vi "object_tracking_subVI_2.vi"(0 "ROI Descriptor (Image Mask 1)":T2={"Global Rectangle"=[272, 198, 466, 320], "Contours"=[{"ID"=enum."External", "Type"=3, "Coordinates"=[272, 198, 466, 320]}]} {"Contours"."Type" items=["No Selection", "Point", "Line", "Rectangle", "Oval", "Polygon", "Freehand Region", "Annulus", "Unused2", "Unused3", "Broken Line", "Freehand Line", "Rotated Rectangle"]}, 1 "Image":T1, 7 "error in":errorcluster) -> (20 "Objects (pixel) (Object Tracking 1)":T3(array[cluster]), 21 "Image Out":T1(plugin-control), 27 "error out":errorcluster)   [LabVIEW 2024]
doc: "Este subVI realiza el procesado de las imágenes capturadas en tiempo real. Contiene el proceso de adquisición, image mask, color plane extraction, gray morphological y object tracking.\n\nAutores:\nIvan Nieto Guerrero, David Alejandro Zarazúa Martínez\n\n06/Mar/2025"
uses:
  <vilib>/vision/Image Controls.llb/IMAQ Image.ctl
  <vilib>/vision/Tracking.llb/IMAQ Object Tracking SessionType.ctl
  <vilib>/vision/Vision Assistant Utils.llb/IVA Object Tracking - Init Function.ctl
  <vilib>/vision/NI_Vision_Development_Module.lvlib
panel:
  in  "error in (no error)":errorcluster
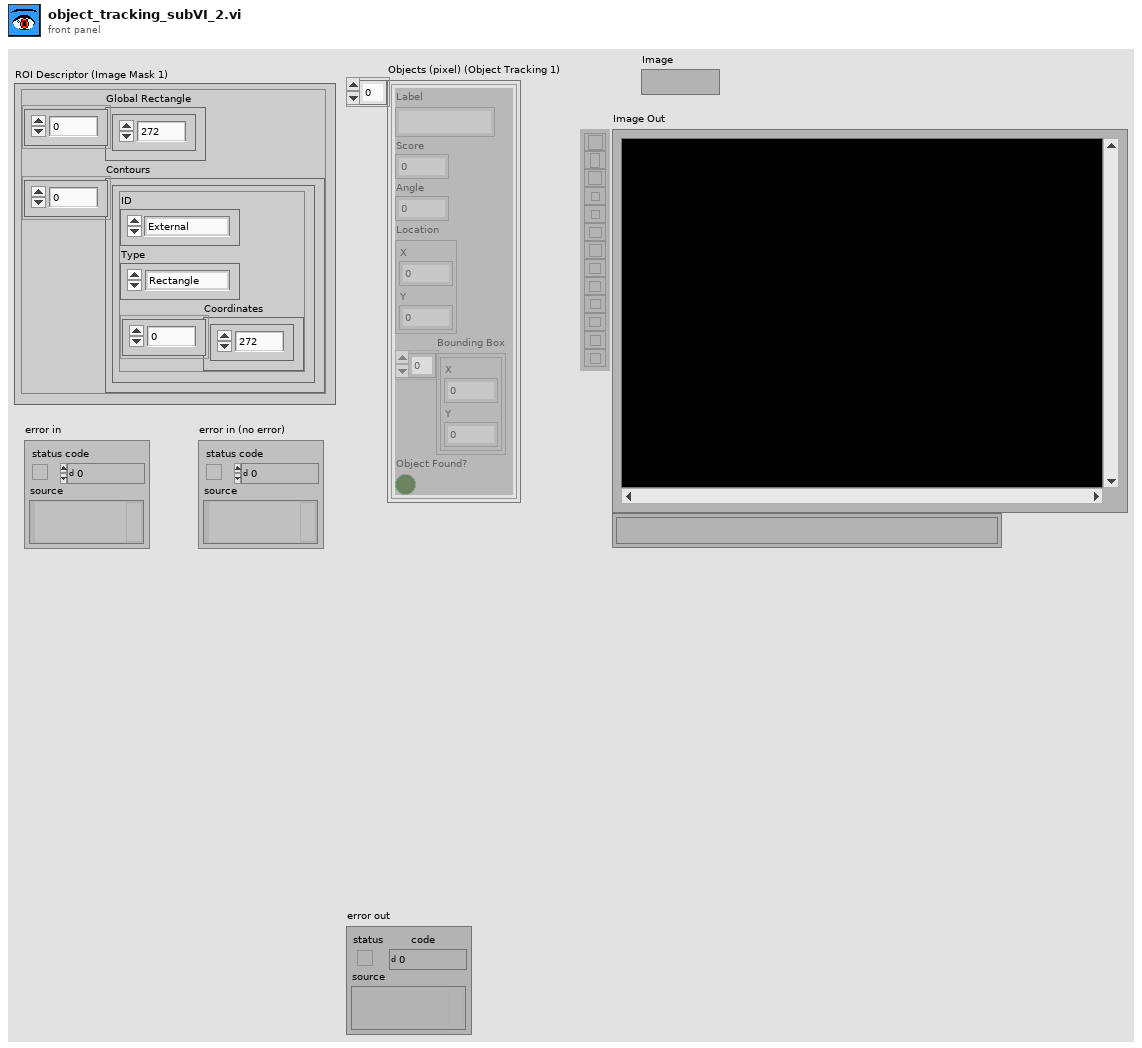
[diagram p1: front panel]
types:
  T1 = typedef "IMAQ Image.ctl" = refnum<image>
  T2 = cluster{"Global Rectangle":i32[], "Contours":cluster{"ID":enum32{"External", "Internal"}, "Type":u32, "Coordinates":i32[]}[]}
  T3 = cluster{"Label":string, "Score":i32, "Angle":dbl, "Location":cluster{"X":dbl, "Y":dbl}, "Bounding Box":cluster{"X":dbl, "Y":dbl}[], "Object Found?":bool}[]
  T4 = cluster{"Number of Histogram Bins":i32, "Blending Parameter (%)":dbl, "Max Scale Change (%)":dbl, "Max Rotation Change":dbl, "Max Shape Change (%)":dbl, "Maximum Iterations":i32}
  T5 = typedef "IVA Object Tracking - Init Function.ctl" = enum16{"Init", "Get", "Set"}
  T6 = cluster{"Initial Position":cluster{"Source":enum16{"Constant", "Measure"}, "Point ID":cluster{"GUID":string, "Index":i32}, "Point":cluster{"x":sgl, "y":sgl}}, "Initial Angle":cluster{"Source":enum16{"Constant", "Measure"}, "Measure ID":cluster{"GUID":string, "Index":i32}, "Value":dbl}}[]
  T7 = typedef "IMAQ Object Tracking SessionType.ctl" = i32
  T8 = enum32{"AutoM", "Close", "Dilate", "Erode", "Gradient", "Gradient in", "Gradient out", "HitMiss", "Open", "PClose", "POpen", "Thick", "Thin"}
  T9 = typedef "Image Type" = u32
  T10 = cluster{"Number of Histogram Bins":i32, "Blending Parameter (%)":dbl, "Maximum Iterations":i32}
  T11 = typedef "IMAQ Object Tracking Session.ctl" = refnum<k20>
  T12 = cluster{"Source":enum16{"Constant", "Measure"}, "Point ID":cluster{"GUID":string, "Index":i32}, "Point":cluster{"x":sgl, "y":sgl}}
  T13 = cluster{"Source":enum16{"Constant", "Measure"}, "Measure ID":cluster{"GUID":string, "Index":i32}, "Value":dbl}
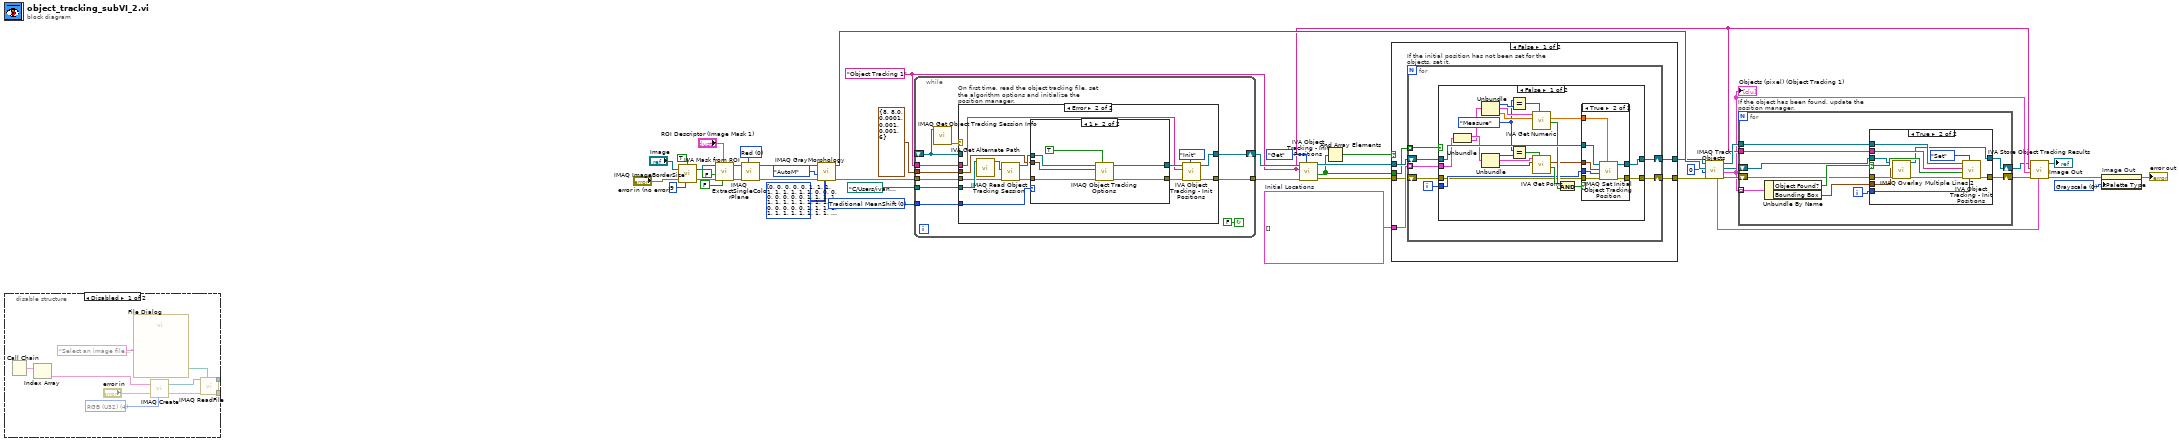
[diagram p0: block diagram]
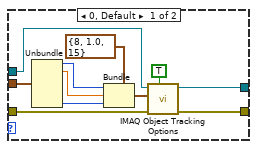
[diagram p8: hidden frame]
diagram:
  w4 = u32 0 items=["Grayscale", "Binary", "Gradient", "Rainbow", "Temperature", "User Defined", "Binary 16 Bit", "Gradient 16 Bit", "Rainbow 16 Bit", "Temperature 16 Bit", "User Defined 16 Bit"] ("Palette Type")
  w12 = "Object Tracking 1" ("Step Name")
  w26 = T6 []  # Initial Locations
  w28 = T7 0 items=["Traditional MeanShift", "Shape Adapted MeanShift"] ("Algorithm")
  w36 = 0 items=["Red", "Green", "Blue", "Hue", "Saturation", "Luminance", "Value", "Intensity"] ("Color Plane")
  n1 = disable-structure shown="Disabled" {
    disable-tunnel: [w54 _] -> _
    disable-tunnel: [w45 _] -> _
    frame Disabled {
      w46 = T9 4 items=["Grayscale (U8)", "Grayscale (I16)", "Grayscale (SGL)", "Complex (CSG)", "RGB (U32)", "HSL (U32)", "RGB (U64)", "Grayscale (U16)"] ("Image Type")
      n2 = Call Chain() -> (call chain=w50:string[])
      n3 = Index Array(array=w50) -> (element=w49:string)  [unwired: 1 in]
      n4 = call "File Dialog"("prompt"="Select an image file...") -> ("selected path"=w47:path)  [unwired: 6 in, 8 out]
      n5 = call "IMAQ Create"("Image Name"=w49, "Image Type"=w46, "error in (no error)"="error in") -> ("New Image"=w53:T1, "error out"=w52:errorcluster)  [unwired: 1 in, 1 out]
      n6 = call "IMAQ ReadFile"("File Path"=w47, "error in (no error)"=w52, "Image"=w53) -> ("error out"=w54:errorcluster, "Image Out"=w45:T1)  [unwired: 2 in, 5 out]
    }
    frame Enabled {
    }
  }
  n7 = call "IMAQ ImageBorderSize"("Get/Set Status? (Set)"=TRUE, "Image"="Image", "Image border size in"=9 ("Border Size"), "error in (no error)"="error in (no error)") -> ("Image Out"=w39:T1, "error out"=w44:errorcluster)  [unwired: 1 out]
  n8 = call <vilib>:"IVA Mask from ROI.vi"("Shrink"=FALSE, "ROI Descriptor"="ROI Descriptor (Image Mask 1)", "error in (no error)"=w44, "Out / In"=FALSE, "Image Src"=w39) -> ("error out"=w37:errorcluster, "Image Out"=w35:T1)  [unwired: 5 out]
  n9 = call "IMAQ ExtractSingleColorPlane"("Color Plane"=w36, "error in (no error)"=w37, "Image Src"=w35) -> ("error out"=w34:errorcluster, "Image Dst Out"=w31:T1)  [unwired: 1 in, 6 out]
  n10 = call "IMAQ GrayMorphology"("Structuring Element"=i32[][] [[0, 0, 0, 0, 0, 1, 1, 1, 1, 1, 1, 1, 1, 1, 0, 0, 0, 0, 0], [0, 0, 0, 1, 1, 1, 1, 1, 1, 1, 1, 1, 1, 1, 1, 1, 0, 0, 0], [0, 0, 1, 1, 1, 1, 1, 1, 1, 1, 1, 1, 1, 1, 1, 1, 1, 0, 0], [0, 1, 1, 1, 1, 1, 1, 1, 1, 1, 1, 1, 1, 1, 1, 1, 1, 1, 0], [0, 1, 1, 1, 1, 1, 1, 1, 1, 1, 1, 1, 1, 1, 1, 1, 1, 1, 0], [1, 1, 1, 1, 1, 1, 1, 1, 1, 1, 1, 1, 1, 1, 1, 1, 1, 1, 1], [1, 1, 1, 1, 1, 1, 1, 1, 1, 1, 1, 1, 1, 1, 1, 1, 1, 1, 1], [1, 1, 1, 1, 1, 1, 1, 1, 1, 1, 1, 1, 1, 1, 1, 1, 1, 1, 1], [1, 1, 1, 1, 1, 1, 1, 1, 1, 1, 1, 1, 1, 1, 1, 1, 1, 1, 1], [1, 1, 1, 1, 1, 1, 1, 1, 1, 1, 1, 1, 1, 1, 1, 1, 1, 1, 1], [1, 1, 1, 1, 1, 1, 1, 1, 1, 1, 1, 1, 1, 1, 1, 1, 1, 1, 1], [1, 1, 1, 1, 1, 1, 1, 1, 1, 1, 1, 1, 1, 1, 1, 1, 1, 1, 1], [1, 1, 1, 1, 1, 1, 1, 1, 1, 1, 1, 1, 1, 1, 1, 1, 1, 1, 1], [1, 1, 1, 1, 1, 1, 1, 1, 1, 1, 1, 1, 1, 1, 1, 1, 1, 1, 1], [0, 1, 1, 1, 1, 1, 1, 1, 1, 1, 1, 1, 1, 1, 1, 1, 1, 1, 0], [0, 1, 1, 1, 1, 1, 1, 1, 1, 1, 1, 1, 1, 1, 1, 1, 1, 1, 0], [0, 0, 1, 1, 1, 1, 1, 1, 1, 1, 1, 1, 1, 1, 1, 1, 1, 0, 0], [0, 0, 0, 1, 1, 1, 1, 1, 1, 1, 1, 1, 1, 1, 1, 1, 0, 0, 0], [0, 0, 0, 0, 0, 1, 1, 1, 1, 1, 1, 1, 1, 1, 0, 0, 0, 0, 0]], "error in (no error)"=w34, "Operation"=T8."AutoM", "Image Src"=w31) -> ("error out"=w30:errorcluster, "Image Dst Out"=w29:T1)  [unwired: 3 in, 3 out]
  n11 = while {
    shift-right: [w64] -> w24
    shift-left: _ -> [w55]
    tunnel: path "C:/Users/ivanu/OneDrive/Escritorio/Universidad/Semestre 8/Instrumentacion/Proyecto Final_Eye_detection/pupila_1.nitf.png" ("Tracking Session File Path") -> [w62]
    tunnel: w30 -> [w61]
    tunnel: w28 -> [w60]
    tunnel: [w59] -> w21
    tunnel: T4 {"Number of Histogram Bins"=8, "Blending Parameter (%)"=8.0, "Max Scale Change (%)"=0.0001, "Max Rotation Change"=0.001, "Max Shape Change (%)"=0.001, "Maximum Iterations"=6} ("Options") -> [w58]
    tunnel: w12 -> [w57]
    stop <- FALSE continue-if-true
    n12 = call "IMAQ Get Object Tracking Session Info"("Object Tracking Session In"=w55) -> ("error out"=w56:errorcluster)  [unwired: 1 in, 9 out]
    n13 = case "On first time, read the object tracking file, set the algorithm options and initialize the position manager." shown="Error" w56 {
      tunnel: [w66 w71] -> w64
      tunnel: w55 -> [w66 _]
      tunnel: w62 -> [_ w79]
      tunnel: w61 -> [w65 w77]
      tunnel: w60 -> [_ w76]
      tunnel: [w65 w70] -> w59
      tunnel: w58 -> [_ w73]
      tunnel: w57 -> [_ w67]
      frame No Error {
      }
      frame Error {
        n14 = call <vilib>:"IVA Get Alternate Path.vi"("Path In"=w79) -> ("Path Out"=w78:path)  [unwired: 10 out]
        n15 = call "IMAQ Read Object Tracking Session"("error in (no error)"=w77, "Object Tracking Session File Path"=w78) -> ("error out"=w74:errorcluster, "Object Tracking Session Out"=w75:T11)  [unwired: 1 in, 7 out]
        n16 = case shown="1" w76 {
          tunnel: w75 -> [w90 w96]
          tunnel: [w89 w95] -> w72
          tunnel: w74 -> [w88 w94]
          tunnel: [w87 w93] -> w69
          tunnel: w73 -> [w86 w92]
          frame 0, Default {
            n17 = Unbundle(w86) -> ("Number of Histogram Bins"=w85:i32, "Blending Parameter (%)"=w84:dbl, "Maximum Iterations"=w80:i32)  [unwired: 3 out]
            n18 = Bundle(cluster=T10 {"Number of Histogram Bins"=8, "Blending Parameter (%)"=1.0, "Maximum Iterations"=15} ("Mean Shift Options in"), "Number of Histogram Bins"=w85, "Blending Parameter (%)"=w84, "Maximum Iterations"=w80) -> (w83:T10)
            n19 = call-poly "IMAQ Object Tracking Options"("Get/Set (Get)"=TRUE, "error in (no error)"=w88, "Mean Shift Options in"=w83, "Object Tracking Session In"=w90) -> ("error out"=w87:errorcluster, "Object Tracking Session Out"=w89:T11)  [unwired: 1 in, 5 out]
          }
          frame 1 {
            n20 = call-poly "IMAQ Object Tracking Options"("Get/Set (Get)"=TRUE, "error in (no error)"=w94, "Shape Adapted Options in"=w92, "Object Tracking Session In"=w96) -> ("error out"=w93:errorcluster, "Object Tracking Session Out"=w95:T11)  [unwired: 2 in, 4 out]
          }
        }
        n21 = call <vilib>:"IVA Object Tracking - Init Positions.vi"("Function"=IVA_Object_Tracking_-_Init_Function."Init", "error in (no error)"=w69, "Process ID"=w67, "Object Tracking Session In"=w72) -> ("error out"=w70:errorcluster, "Object Tracking Session dup"=w71:T11)  [unwired: 2 in, 4 out]
      }
    }
  }
  n22 = call <vilib>:"IVA Object Tracking - Init Positions.vi"("Function"=IVA_Object_Tracking_-_Init_Function."Get", "error in (no error)"=w21, "Process ID"=w12, "Object Tracking Session In"=w24) -> ("error out"=w20:errorcluster, "Init Values Out"=w18:bool[], "Object Tracking Session dup"=w23:T11)  [unwired: 2 in, 3 out]
  n23 = And Array Elements(Boolean array=w18) -> (logical AND=w19:bool)
  n24 = case shown="False" w19 {
    tunnel: w26 -> [w102 _]
    tunnel: [w101 w144] -> w25
    tunnel: w23 -> [w100 w144]
    tunnel: w20 -> [w99 w143]
    tunnel: w18 -> [w98 _]
    tunnel: [w97 w143] -> w17
    frame False {
      n25 = for "If the initial position has not been set for the objects, set it." {
        tunnel: w102 -> [w108] mode=indexing
        shift-right: [w106] -> w101
        shift-left: w100 -> [w109]
        shift-right: [w103] -> w97
        shift-left: w99 -> [w105]
        tunnel: w98 -> [w104] mode=indexing
        i -> [w107]
        n26 = case shown="False" w104 {
          tunnel: w109 -> [w131 w142]
          tunnel: w108 -> [w130 _]
          tunnel: w107 -> [w114 _]
          tunnel: [w112 w142] -> w106
          tunnel: w105 -> [w111 w141]
          tunnel: [w110 w141] -> w103
          frame False {
            w120 = enum16{"Constant", "Measure"}."Measure" ("Source")
            n27 = Unbundle(w130) -> ("Initial Position"=w129:T12, "Initial Angle"=w128:T13)
            n28 = Unbundle(w128) -> ("Source"=w121:enum16{"Constant", "Measure"}, "Measure ID"=w125:cluster{"GUID":string, "Index":i32}, "Value"=w124:dbl)
            n29 = Unbundle(w129) -> ("Source"=w123:enum16{"Constant", "Measure"}, "Point ID"=w127:cluster{"GUID":string, "Index":i32}, "Point"=w126:cluster{"x":sgl, "y":sgl})
            n30 = Equal?(x=w120, y=w121) -> (x = y?=w119:bool)
            n31 = Equal?(x=w120, y=w123) -> (x = y?=w122:bool)
            n32 = call <vilib>:"IVA Get Numeric.vi"("Source"=w119, "Numeric in"=w124, "Result ID"=w125) -> ("Available?"=w117:bool, "Numeric out"=w113:dbl)  [unwired: 1 in, 6 out]
            n33 = call <vilib>:"IVA Get Point.vi"("Point Source"=w122, "Point in"=w126, "Point ID"=w127) -> ("Available?"=w118:bool, "Point out"=w115:cluster{"x":sgl, "y":sgl})  [unwired: 1 in, 6 out]
            n34 = And(x=w118, y=w117) -> (x .and. y?=w116:bool)
            n35 = case shown="True" w116 {
              tunnel: w131 -> [w133 w140]
              tunnel: w115 -> [_ w139]
              tunnel: w114 -> [_ w138]
              tunnel: w113 -> [_ w134]
              tunnel: [w133 w137] -> w112
              tunnel: w111 -> [w132 w136]
              tunnel: [w132 w135] -> w110
              frame False {
              }
              frame True {
                n36 = call "IMAQ Set Initial Object Tracking Position"("Initial Angle"=w134, "error in (no error)"=w136, "Object Index"=w138, "Position"=w139, "Object Tracking Session In"=w140) -> ("error out"=w135:errorcluster, "Object Tracking Session Out"=w137:T11)  [unwired: 5 out]
              }
            }
          }
          frame True {
          }
        }
      }
    }
    frame True {
    }
  }
  n37 = call "IMAQ Track Objects"("error in (no error)"=w17, "Minimum Score"=0, "Image"=w29, "Object Tracking Session In"=w25) -> ("error out"=w16:errorcluster, "Objects (pixel)"=w11:T3, "Image (duplicate)"=w8:T1, "Object Tracking Session Out"=w15:T11, "Objects (real-world)"=w10:T3)  [unwired: 3 out]
  "Objects (pixel) (Object Tracking 1)" <- w11
  n38 = for "If the object has been found, update the position manager." {
    tunnel: w11 -> [w154] mode=indexing
    tunnel: w12 -> [w153]
    shift-right: [w150] -> w14
    shift-left: w16 -> [w147]
    tunnel: w15 -> [w152]
    shift-right: [w146] -> w7
    shift-left: w8 -> [w148]
    i -> [w149]
    n39 = Unbundle By Name(w154) -> ("Object Found?"=w151:bool, "Bounding Box"=w145:cluster{"X":dbl, "Y":dbl}[])
    n40 = case shown="True" w151 {
      selector: w151 -> [_ w164]
      tunnel: w153 -> [_ w166]
      tunnel: w152 -> [_ w165]
      tunnel: [w156 w163] -> w150
      tunnel: w149 -> [_ w162]
      tunnel: w148 -> [w155 w161]
      tunnel: w147 -> [w156 w159]
      tunnel: [w155 w158] -> w146
      tunnel: w145 -> [_ w157]
      frame False {
      }
      frame True {
        n41 = call "IMAQ Overlay Multiple Lines 2"("Image"=w161, "Line End Points"=w157, "error in (no error)"=w159) -> ("Image Out"=w158:T1, "error out"=w160:errorcluster)  [unwired: 11 in]
        n42 = call <vilib>:"IVA Object Tracking - Init Positions.vi"("Index"=w162, "Function"=IVA_Object_Tracking_-_Init_Function."Set", "error in (no error)"=w160, "Value"=w164, "Process ID"=w166, "Object Tracking Session In"=w165) -> ("error out"=w163:errorcluster)  [unwired: 5 out]
      }
    }
  }
  n43 = call <vilib>:"IVA Store Object Tracking Results.vi"("Objects (real-world)"=w10, "error in (no error)"=w14, "Objects (pixel)"=w11, "Step Name"=w12, "Image in"=w7) -> ("error out"=w13:errorcluster, "Image dup"=→"Image Out":T1)  [unwired: 5 out]
  n44 = property on="Image Out" class="ImageControl"(error in=w13, "Palette:Palette Type"=w4) -> (error out=→"error out":errorcluster)  [unwired: 1 in, 1 out]
